vi "zadanie_2.vi"() -> ()   [LabVIEW 2020]
panel:
  out "Sekundy":dbl
  out "Minuty":dbl
  out "Godziny":dbl
  in  "Całkowity czas w sekundach":dbl
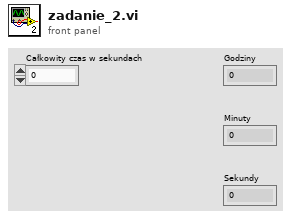
[diagram p1: front panel]
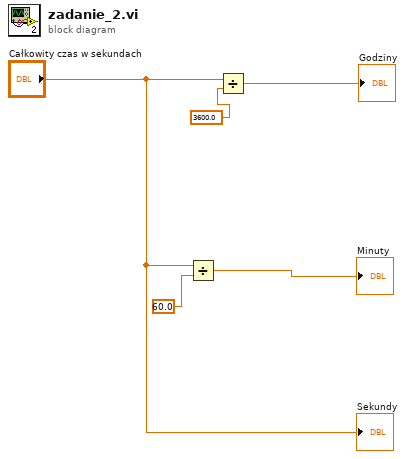
[diagram p0: block diagram]
diagram:
  n1 = Divide(x="Całkowity czas w sekundach", y=60.0) -> (x/y=→"Minuty":dbl)
  n2 = Divide(x="Całkowity czas w sekundach", y=3600.0) -> (x/y=→"Godziny":dbl)
  "Sekundy" <- "Całkowity czas w sekundach"
